vi "Get Operator Name.vi"(10 "error in (no error)":errorcluster) -> (2 "error out":errorcluster, 5 "Operator Name":string)   [LabVIEW 2017]
uses:
  Database/Controls/DB Options.ctl
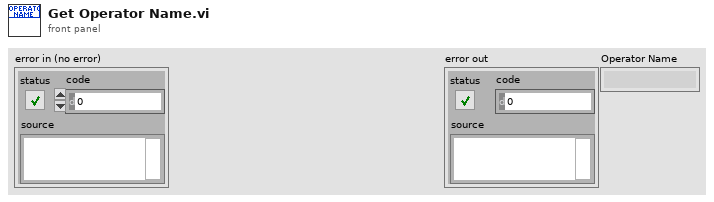
[diagram p1: front panel]
types:
  T1 = typedef "DB Options.ctl" = enum16{"Select", "Execute", "Special Q", "Insert", "Update", "Delete", "Open", "Close"}
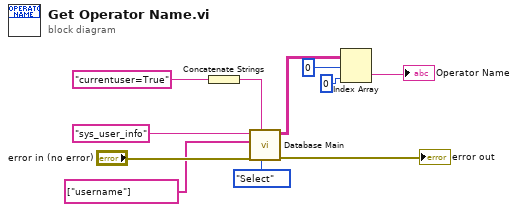
[diagram p0: block diagram]
diagram:
  n1 = Concatenate Strings("currentuser=True" ("string")) -> (w6:string)
  n2 = call "Database Main.vi"("Option"=DB_Options."Select", "Where"=w6, "error in (no error)"="error in (no error)", "Column Name"=string[] ["username"], "table Name/Query"="sys_user_info") -> ("error out"=→"error out":errorcluster, "Data"=w9:string[][])  [unwired: 4 in, 1 out]
  n3 = Index Array(array=w9, index (row)=0 ("disabled index (row)"), index (col)=0) -> (element=→"Operator Name":string)
